vi "ReconocimientoVoz (SubVI).vi"(10 "Sensibility":dbl) -> (1 "similarities":cdb[](array[numeric]), 2 "hasAccess":bool, 3 "AudioRecorded":waveform(dbl)[](graph), 4 "Name":string)   [LabVIEW 2017]
uses:
  <vilib>/Analysis/NI_AALPro.lvlib
  <vilib>/Analysis/2dsp.llb/1D Cross Correlation (DBL).vi
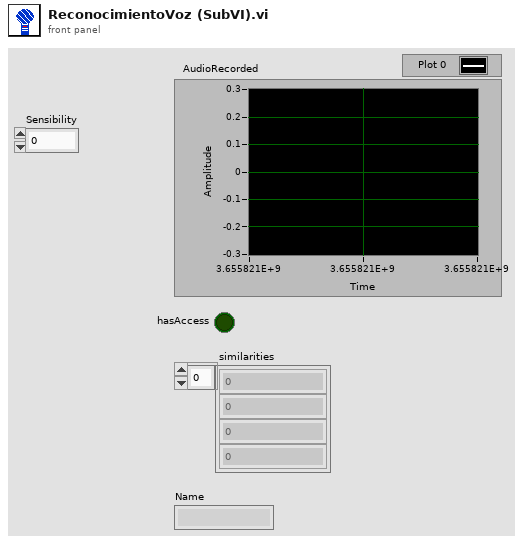
[diagram p1: front panel]
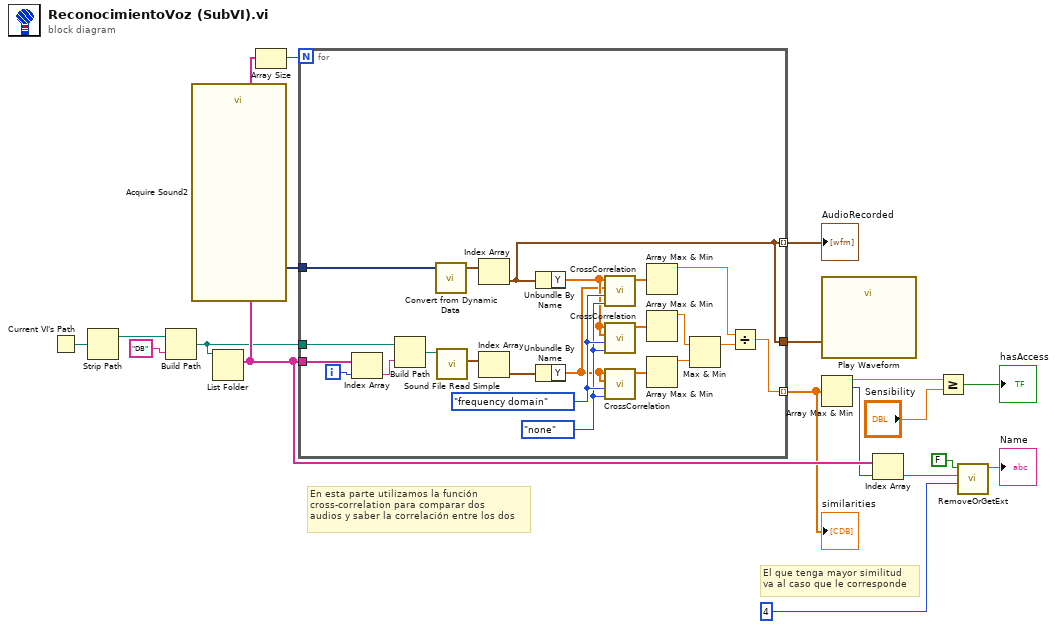
[diagram p0: block diagram]
diagram:
  # "El que tenga mayor similitud\nva al caso que le corresponde"
  # "En esta parte utilizamos la función\ncross-correlation para comparar dos\naudios y saber la correlación entre los dos"
  n1 = Current VI's Path() -> (path=w5:path)
  n2 = Strip Path(path=w5) -> (stripped path=w4:path)  [unwired: 1 out]
  n3 = Build Path(base path=w4, name or relative path="DB") -> (appended path=w2:path)
  n4 = call "Acquire Sound2"() -> ("Data"=w1:dynamicdata)  [unwired: 18 in, 1 out]
  n5 = List Folder(path=w2) -> (filenames=w15:string[])  [unwired: 3 in, 3 out]
  n6 = Array Size(array=w15) -> (size(s)=w11:i32)
  n7 = for {
    N: w11 -> [_]
    tunnel: [w28] -> w10 mode=indexing
    tunnel: [w23] -> w13
    tunnel: w15 -> [w27]
    tunnel: [w23] -> w12 mode=indexing
    tunnel: w1 -> [w21]
    tunnel: w2 -> [w19]
    i -> [w26]
    w40 = enum32{"direct", "frequency domain"}."frequency domain" ("algorithm")
    w39 = enum32{"none", "unbiased", "biased"}."none" ("normalization")
    n8 = Index Array(array=w27, index=w26) -> (element=w25:string)
    n9 = Build Path(base path=w19, name or relative path=w25) -> (appended path=w24:path)
    n10 = call "Convert from Dynamic Data"("Dynamic Data Type"=w21) -> ("Array of Waveform"=w20:waveform(dbl)[])  [unwired: 3 in]
    n11 = call <vilib>:"Sound File Read Simple.vi"("path"=w24) -> ("data"=w30:waveform(dbl)[])  [unwired: 7 in, 3 out]
    n12 = Index Array(array=w20) -> (element=w23:waveform(dbl))  [unwired: 1 in]
    n13 = Index Array(array=w30) -> (element=w22:waveform(dbl))  [unwired: 1 in]
    n14 = Unbundle By Name(w23) -> ("Y"=w31:dbl[])
    n15 = Unbundle By Name(w22) -> ("Y"=w29:dbl[])
    n16 = call-poly <vilib>:"CrossCorrelation.vi"("normalization"=w39, "algorithm"=w40, "Y"=w29, "X"=w31) -> ("Rxy"=w36:dbl[])  [unwired: 6 in, 1 out]
    n17 = call-poly <vilib>:"CrossCorrelation.vi"("normalization"=w39, "algorithm"=w40, "Y"=w31, "X"=w31) -> ("Rxy"=w35:dbl[])  [unwired: 6 in, 1 out]
    n18 = call-poly <vilib>:"CrossCorrelation.vi"("normalization"=w39, "algorithm"=w40, "Y"=w29, "X"=w29) -> ("Rxy"=w34:dbl[])  [unwired: 6 in, 1 out]
    n19 = Array Max & Min(array=w36) -> (max value=w38:dbl)  [unwired: 3 out]
    n20 = Array Max & Min(array=w35) -> (max value=w32:dbl)  [unwired: 3 out]
    n21 = Array Max & Min(array=w34) -> (max value=w33:dbl)  [unwired: 3 out]
    n22 = Max & Min(x=w32, y=w33) -> (max(x,y)=w37:dbl)  [unwired: 1 out]
    n23 = Divide(x=w38, y=w37) -> (x/y=w28:dbl)
  }
  "similarities" <- w10
  "AudioRecorded" <- w12
  n24 = call "Play Waveform"("Data"=w13) -> ()  [unwired: 18 in, 1 out]
  n25 = Array Max & Min(array=w10) -> (max value=w16:dbl, max index (indices)=w14:i32)  [unwired: 2 out]
  n26 = Index Array(array=w15, index=w14) -> (element=w9:string)
  n27 = Greater Or Equal?(x=w16, y="Sensibility") -> (x >= y?=→"hasAccess":bool)
  n28 = call "RemoveOrGetExt.vi"("Longitud de la cadena"=4, "String in"=w9, "Extension-T-Nombre-F"=FALSE) -> ("String out"=→"Name":string)  [unwired: 8 in]
